vi "First Step.vi"(8 "error in (no error)":errorcluster, 11 "Magnetic Field.lvclass in":refnum<class "Magnetic Field.lvclass">) -> (0 "error out":errorcluster, 2 "Current Position":dbl, 3 "Magnetic Field.lvclass out":refnum<class "Magnetic Field.lvclass">)   [LabVIEW 2009, in "Magnetic Field.lvclass"]
uses:
  Magnetic Field.lvclass
  Scanner/Scanner.lvclass
  Instruments/Magnet/Magnet.lvclass
panel:
  out "persis?":bool caption="Persistent"
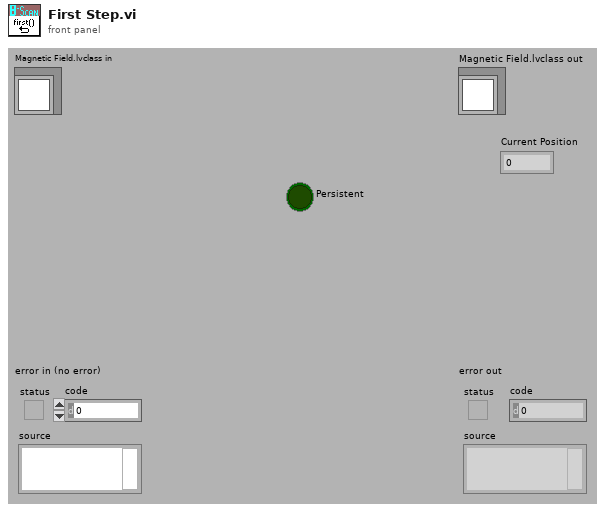
[diagram p1: front panel]
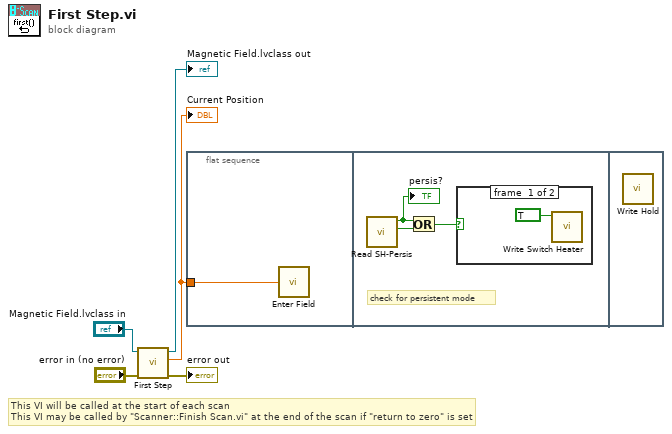
[diagram p0: block diagram]
diagram:
  # "This VI will be called at the start of each scan\nThis VI may be called by \"Scanner::Finish Scan.vi\" at the end of the scan if \"return to zero\" is set"
  n1 = call-parent "First Step.vi"("error in (no error)"="error in (no error)", "Scanner.lvclass in"="Magnetic Field.lvclass in") -> ("error out"=→"error out":errorcluster, "Current Position"=w1:dbl, "Scanner.lvclass out"=→"Magnetic Field.lvclass out":refnum<class "Magnetic Field.lvclass">)  [unwired: 7 out]
  "Current Position" <- w1
  n2 = flat-sequence {
    tunnel: w1 -> [w6]
    frame #0 {
      n3 = call "Enter Field.vi"("field"=w6) -> ()  [unwired: 2 in, 3 out]
    }
    frame #1 {
      # "check for persistent mode"
      n4 = call "Read SH-Persis.vi"() -> ("pers?"=w7:bool, "SHon?"=w8:bool)  [unwired: 5 out]
      "persis?" <- w7
      n5 = Or(x=w7, y=w8) -> (x .or. y?=w9:bool)
      n6 = case shown="False" w9 {
        frame #0 {
          n7 = call "Write Switch Heater.vi"("switchheater"=TRUE) -> ()  [unwired: 7 out]
        }
        frame #1 {
        }
      }
    }
    frame #2 {
      n8 = call "Write Hold.vi"() -> ()  [unwired: 8 out]
    }
  }
